vi "face reverserows.vi"(8 "error in (no error)":errorcluster, 11 "face in":T1) -> (0 "error out":errorcluster, 3 "face out":T1)   [LabVIEW 2011]
uses:
  Typedef/face.ctl
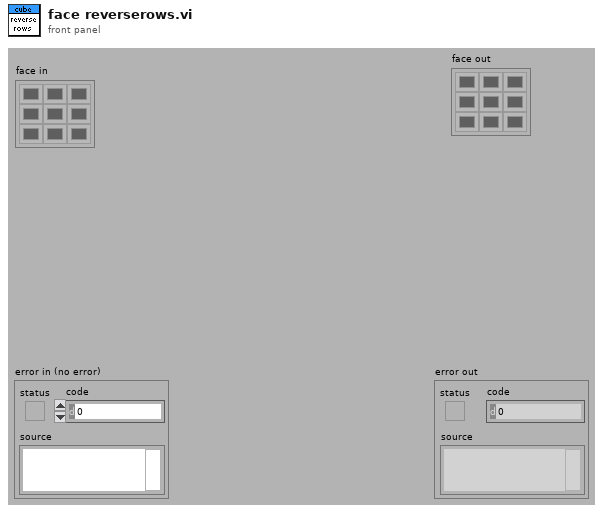
[diagram p1: front panel]
types:
  T1 = typedef "face.ctl" = u32[][]
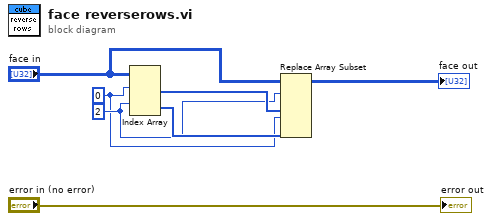
[diagram p0: block diagram]
diagram:
  w2 = 2 ("index (col)")
  w1 = 0 ("disabled index (col)")
  n1 = Index Array(array="face in", index (row) #1=w1, index (row) #2=w2) -> (element #1=w5:u32[], element #2=w4:u32[])  [unwired: 2 in]
  n2 = Replace Array Subset(array="face in", new element #1=w5, index (row) #1=w2, new element #2=w4, index (row) #2=w1) -> (→"face out":T1)  [unwired: 2 in]
  "error out" <- "error in (no error)"
